vi "Untitled 3.vi"() -> ()   [LabVIEW 2016]
uses:
  <vilib>/Utility/miscctls.llb/LV3DPointTypeDef.ctl
  <vilib>/picture/3D Picture Control/Object/Create Object (drawable).vi
  <vilib>/picture/3D Picture Control/Object/Add Object (no reference).vi
  <vilib>/picture/3D Picture Control/NI_3D Picture Control.lvlib
panel:
  in  "Up Direction":T1
  in  "Target":T1
  in  "Camera Position":T1
  in  "Stop Button":bool
  out "3D Picture":refnum<vi>(3d-picture)
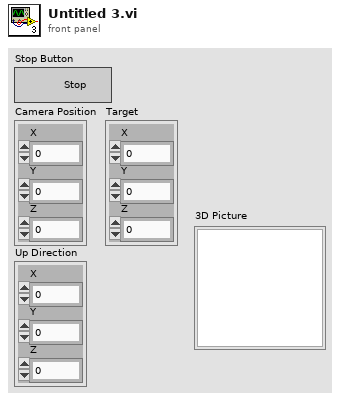
[diagram p1: front panel]
types:
  T1 = typedef "LV3DPointTypeDef.ctl" = cluster{"X":sgl, "Y":sgl, "Z":sgl}
  T2 = cluster{"number: 0 to 1":dbl, "number: 0 to 1":dbl, "number: 0 to 1":dbl}
  T3 = cluster{"number: 0 to 1":dbl, "number: 0 to 1":dbl, "number: 0 to 1":dbl, dbl}
  T4 = enum16{"Overall", "Per Primitive", "Per Vertex", "Binding Off"}
  T5 = enum16{"Points", "Lines", "Line Strip", "Line Loop", "Triangles", "Triangle Strip", "Triangle Fan", "Quads", "Quad Strip", "Polygon"}
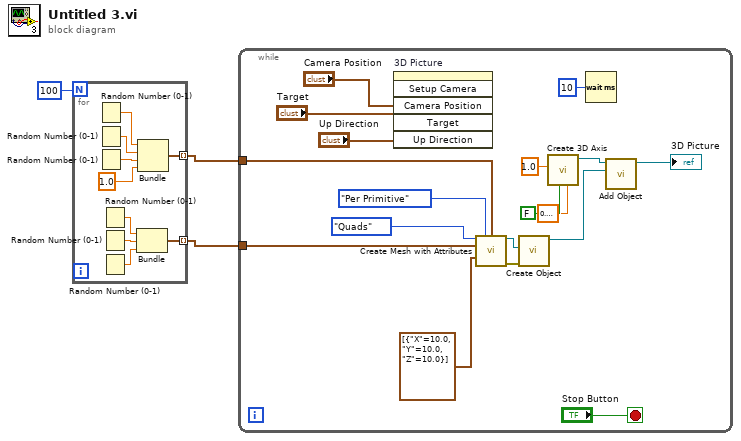
[diagram p0: block diagram]
diagram:
  n1 = for {
    N: 100 -> [_]
    tunnel: [w6] -> w2 mode=indexing
    tunnel: [w5] -> w3 mode=indexing
    n2 = Random Number (0-1)() -> (number: 0 to 1=w12:dbl)
    n3 = Random Number (0-1)() -> (number: 0 to 1=w10:dbl)
    n4 = Random Number (0-1)() -> (number: 0 to 1=w11:dbl)
    n5 = Random Number (0-1)() -> (number: 0 to 1=w7:dbl)
    n6 = Random Number (0-1)() -> (number: 0 to 1=w9:dbl)
    n7 = Random Number (0-1)() -> (number: 0 to 1=w8:dbl)
    n8 = Bundle("number: 0 to 1"=w7, "number: 0 to 1"=w9, "number: 0 to 1"=w8) -> (w6:T2)  [unwired: 1 in]
    n9 = Bundle("number: 0 to 1"=w12, "number: 0 to 1"=w10, "number: 0 to 1"=w11, 1.0) -> (w5:T3)  [unwired: 1 in]
  }
  n10 = while {
    tunnel: w3 -> [w23]
    tunnel: w2 -> [w22]
    stop <- "Stop Button" stop-if-true
    n11 = invoke on="3D Picture" class="SceneGraphDisp (strict)" method="Setup Camera"("Camera Position"="Camera Position", "Target"="Target", "Up Direction"="Up Direction") -> ()  [unwired: 3 in, 6 out]
    n12 = call <vilib>:"Create Mesh with Attributes.vi"("Draw Mode"=T5."Quads", "Color Binding Mode"=T4."Per Primitive", "Color Array"=w23, "Vertex Array"=w22, "Normal Array"=cluster{"X":sgl, "Y":sgl, "Z":sgl}[] [{"X"=10.0, "Y"=10.0, "Z"=10.0}]) -> ("New Mesh Refnum"=w27:refnum<vi>, "error out"=w28:errorcluster)  [unwired: 9 in]
    n13 = call-poly <vilib>:"Create Object.vi"("error in (no error)"=w28, "Geometry"=w27) -> ("Scene:New Object"=w14:refnum<vi>)  [unwired: 8 in, 1 out]
    n14 = call <vilib>:"Create 3D Axis.vi"("Character Size"=sgl 0.2, "Axis label?"=FALSE, "Length"=sgl 1.0) -> ("New Object Refnum"=w15:refnum<vi>)  [unwired: 7 in, 1 out]
    n15 = Wait (ms)(milliseconds to wait=u32 10) -> ()  [unwired: 1 out]
    n16 = call-poly <vilib>:"Add Object.vi"("New Object In"=w14, "Scene Object In"=w15) -> ("Scene Object Out"=→"3D Picture":refnum<vi>)  [unwired: 8 in, 1 out]
  }
